vi "FTW-Test-JSON-NumberFormats.vi"() -> ()   [LabVIEW 2015]
uses:
  source/container/FTW-Container.lvclass
panel:
  out "String 3":string
  out "x = y?":bool
  out "String 2":string
  out "error out":errorcluster
  in  "String":string="[\n    -9223372036854775808,\n    -2147483648,\n    -32768,\n    -128,\n    0,\n    255,\n    256,\n    65535,\n    65536,\n    2147483647,\n    2147483648,\n    9223372036854775807,\n    9223372036854775808,\n    0.1,\n    1.2,\n    1.23,\n    1.234,\n    1.2345,\n    1.23456,\n    1.234567,\n    1.2345678,\n    1.23456789,\n    1.234567899,\n    1.2345678901,\n    1.23456789012,\n    1.234567890123,\n    1.2345678901234,\n    1.23456789012345,\n    1.234567890123456,\n    1.2345678901234567,\n    1.23456789012345678,\n    1.234567890123456789,\n    1.2345678901234567899,\n    1.23456789012345678901,\n    1.234567890123456789012,\n    1.2345678901234567890123,\n    1.23456789012345678901234,\n    1.234567890123456789012345,\n    1.2345678901234567890123456,\n    1.23456789012345678901234567,\n    1.234567890123456789012345678,\n    1.2345678901234567890123456789,\n    1.23456789012345678901234567899,\n    1.234567890123456789012345678901,\n    1.2345678901234567890123456789012,\n    1.23456789012345678901234567890123,\n    1.234567890123456789012345678901234,\n    1.2345678901234567890123456789012345,\n    1.23456789012345678901234567890123456,\n    1.234567890123456789012345678901234567,\n    1.2345678901234567890123456789012345678,\n    1.23456789012345678901234567890123456789,\n    1.234567890123456789012345678901234567899\n]"
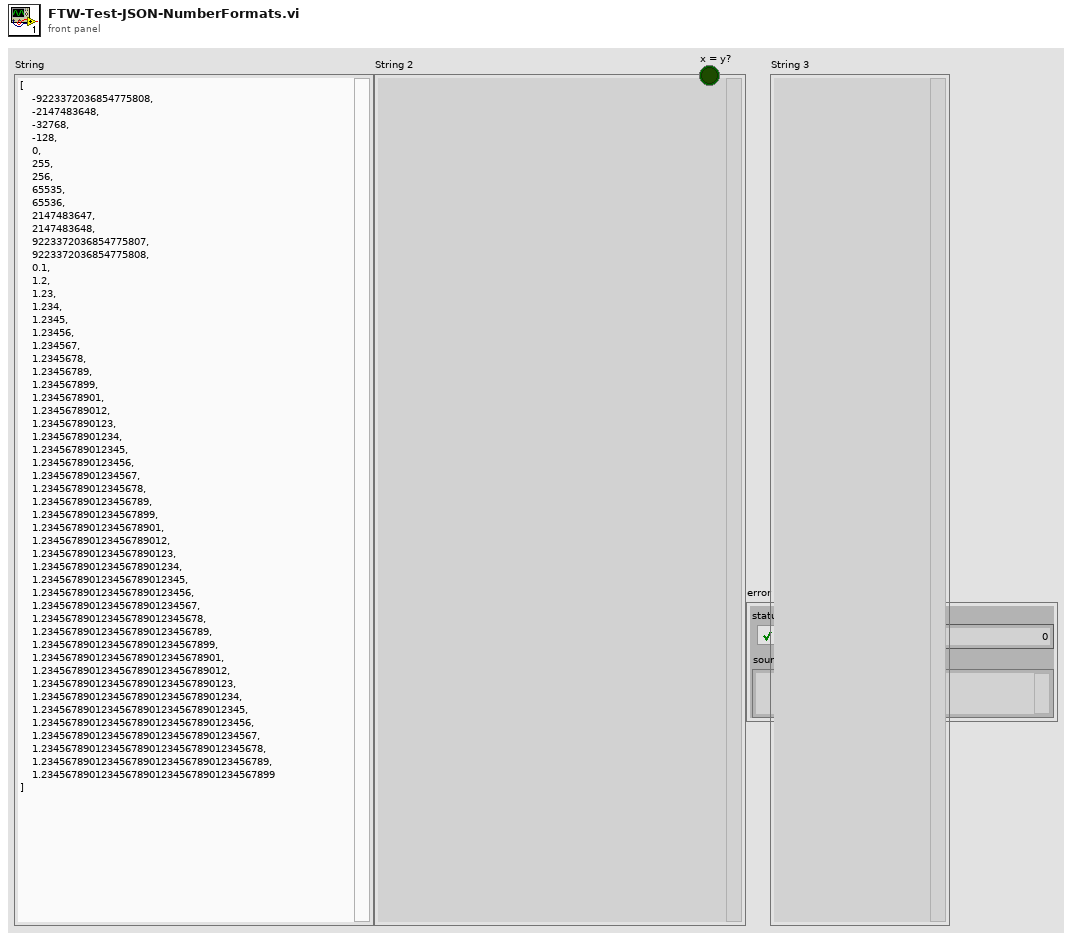
[diagram p1: front panel]
types:
  T1 = typedef "FTW-Container.lvclass/FTW-Container-Type.ctl" = enum8{"invalid", "String", "Integer", "Real", "Object", "Array", "Boolean", "null"}
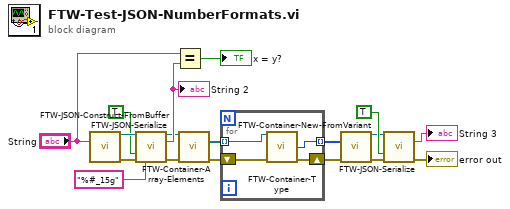
[diagram p0: block diagram]
diagram:
  n1 = call "FTW-JSON-Construct-FromBuffer.vi"("JSON String (UTF-8)"="String") -> ("JSON"=w16:refnum<class "FTW-Container.lvclass">, "error out"=w18:errorcluster)  [unwired: 13 in]
  n2 = call "FTW-JSON-Serialize.vi"("JSON"=w16, "Pretty Print"=TRUE, "error in"=w18, "Real Format"="%#_15g") -> ("JSON out"=w10:refnum<class "FTW-Container.lvclass">, "JSON String (UTF-8)"=w13:string, "error out"=w17:errorcluster)  [unwired: 9 in]
  "String 2" <- w13
  n3 = Equal?(x="String", y=w13) -> (x = y?=→"x = y?":bool)
  n4 = call "FTW-Container-Array-Elements.vi"("FTW-Container In"=w10, "error in"=w17) -> ("Array Elements"=w9:refnum<class "FTW-Container.lvclass">[], "error out"=w11:errorcluster)  [unwired: 11 in, 1 out]
  n5 = for {
    tunnel: w9 -> [w20] mode=indexing
    shift-right: [w21] -> w7
    shift-left: w11 -> [w22]
    tunnel: [w19] -> w8 mode=indexing
    n6 = call "FTW-Container-Type.vi"("FTW-Container In"=w20, "error in"=w22) -> ("Type"=w19:T1, "error out"=w21:errorcluster)  [unwired: 11 in, 1 out]
  }
  n7 = call "FTW-Container-New-FromVariant.vi"("Variant"=w8, "error in"=w7) -> ("FTW-Container"=w5:refnum<class "FTW-Container.lvclass">, "error out"=w4:errorcluster)  [unwired: 12 in]
  n8 = call "FTW-JSON-Serialize.vi"("JSON"=w5, "Pretty Print"=TRUE, "error in"=w4) -> ("JSON String (UTF-8)"=→"String 3":string, "error out"=→"error out":errorcluster)  [unwired: 10 in, 1 out]
